vi "Scale Array.vi"(10 "Scaling Info":T1, 11 "Array to Scale":dbl[](array[numeric])) -> (3 "Scaled Array":dbl[](array[numeric]))   [LabVIEW 2015, in "Neural Network.lvclass"]
doc: "Apply scaling to input vector."
uses:
  Neural Network.lvclass
  Types/Scaling Info.ctl
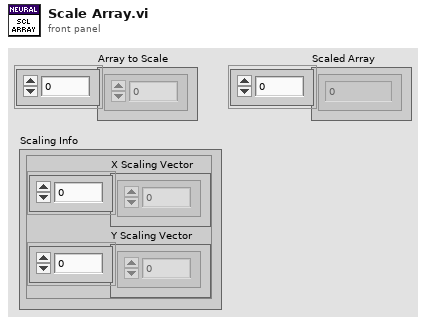
[diagram p1: front panel]
types:
  T1 = typedef "Neural Network.lvclass/Scaling Info.ctl" = cluster{"X Scaling Vector":dbl[], "Y Scaling Vector":dbl[]}
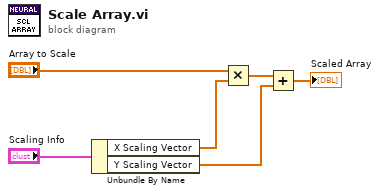
[diagram p0: block diagram]
diagram:
  n1 = Unbundle By Name("Scaling Info") -> ("X Scaling Vector"=w2:dbl[], "Y Scaling Vector"=w1:dbl[])
  n2 = Multiply(x="Array to Scale", y=w2) -> (x*y=w5:dbl[])
  n3 = Add(x=w5, y=w1) -> (x+y=→"Scaled Array":dbl[])
